vi "2ndStrikerV1.vi"(0 "command\nenum":T11, 1 "Toral de n\natacantes":i32, 2 "Total de robos":u32[](array[numeric]), 3 "N atacantes":u32[](array[numeric]), 4 "AI Parameters":T1={"GotoKick"={"Dist do cone a frente"=150.0, "attacker farback"=1500.0, "Perto"=300.0, "min dist to kick"=150.0, "kick eps"=0.0, "Time to transition"=0.05}, "Attacker"={"CC chute"=0.09, "CC passe"=0.045, "Kick Force"=100.0, "ball-robot Kick"=200.0, "ball-robot Pass"=0.3, "drible\nAttk"=FALSE}, "Defender"={"D max"=1700.0, "Vel p/ robô av"=1000.0, "Kick Force"=100.0, "D atk-def"=0.0, "D farback"=0.0, "drible\ndef"=FALSE, "drible\ngoalie"=FALSE}, "Timeout"={"Field/v in x"=6.0, "Dist Robots"=300, "Dist up in y"=300}, "Pose Striker"={"dist"=200.0, "Numeric"=-4.0, "dist 2"=200.0, "drible\nstriker"=FALSE}, "Dist Stop"=300.0, "D ball out"=200, "D central gap "=150.0, "T pass"=0.0, "Force ++"=0.0, "range kick"=0.0, "Chute alto"=TRUE, "Marcador novo"=TRUE, "drible"=FALSE, "D drible"=300.0, "Versão Striker"=enum."3", "Defesa"=enum."ManMark", "Marcador"=enum."Marcar Segndo mais perigoso", "Receptor passe"=enum."2nd Striker", "Área"=enum."Quadrada"} {"D drible" format="%#_13g"; "D central gap" format="%#_13g"; "Dist Stop" format="%#_13g"; "Pose Striker"."Numeric" format="%#_13g"; "Defender"."Kick Force" format="%#_13g"; "Defender"."Vel p/ robô av" format="%#_13g"; "Attacker"."ball-robot Kick" format="%#_13g"; "Attacker"."Kick Force" format="%#_13g"; "Attacker"."CC passe" format="%#_13g"; "Attacker"."CC chute" format="%#_13g"; "GotoKick"."kick eps" format="%#_13g"; "GotoKick"."min dist to kick" format="%#_13g"; "GotoKick"."Perto" format="%#_13g"; "GotoKick"."attacker farback" format="%#_13g"; "GotoKick"."Dist do cone a frente" format="%#_13g"}, 5 "Robot":T2={"id"=0, "function"=enum."Attacker", "x"=0.0, "y"=0.0, "orientation"=0.0, "v_tangent"=0.0, "v_normal"=0.0, "v_ang"=0.0, "kick_x"=0.0, "kick_z"=0.0, "dribble"=FALSE, "Timestamp"=timestamp(0 s since 1904-01-01), "estimatives"={"est_v_tangent"=0.0, "est_v_normal"=0.0, "est_vx"=0.0, "est_vy"=0.0, "Pos Robot Est"=[]}, "dest_x_kick"=0.0, "dest_y_kick"=0.0, "Gap Coord"=[], "States"=enum."GoToTangent", "Path "=[], "Path  Smooth"=[], "Dest"=[]}, 7 "Field defense":dbl[](array[numeric]), 9 "IA Input":T7={"our_robots"=[], "enemy_robots"=[], "balls"=[], "geometry"={"line_width"=0, "field_length"=0, "field_width"=0, "boundary_width"=0, "referee_width"=0, "goal_width"=0, "goal_depth"=0, "goal_wall_width"=0, "center_circle_radius"=0, "defense_radius"=0, "defense_stretch"=0, "free_kick_from_defense_dist"=0, "penalty_spot_from_field_line_dist"=0, "penalty_line_from_spot_dist"=0}, "IA Judge"={"stage"="", "command"="", "our_goalie_id"=0.0, "enemy_goalie_id"=0.0, "command enum"=enum."Halt", "Time"=enum."Azul"}, "Received Timestamp"=timestamp(0 s since 1904-01-01), "Events"={"Touch"=FALSE, "Ball out"=FALSE, "id touch"=0.0, "Ball out of \nVision"=FALSE, "Ball inside \nGoalie area"=FALSE, "Robot not responding"=FALSE, "Robots responding status"=[1.0, 1.0, 1.0, 1.0, 1.0, 1.0], "Enemy Ball \nPossession"=FALSE, "Pass State"=FALSE, "id end of pass"=0.0, "Kick"=FALSE, "Id ini Possession"=0.0, "Ball Possesion"=FALSE, "Id Possesion"=0.0, "Direct Kick"=FALSE, "2nd Strk Ativo"=FALSE}}, 11 "atacando ao contrário?":bool=TRUE, 12 "Impulso de\ntime elapsed":bool=TRUE, 13 "geometry":T9, 14 "balls":T8[](array[typedef]), 15 "Início de pass state":bool=TRUE) -> (6 "Robot out":T2={"id"=0, "function"=enum."Attacker", "x"=0.0, "y"=0.0, "orientation"=0.0, "v_tangent"=0.0, "v_normal"=0.0, "v_ang"=0.0, "kick_x"=0.0, "kick_z"=0.0, "dribble"=FALSE, "Timestamp"=timestamp(0 s since 1904-01-01), "estimatives"={"est_v_tangent"=0.0, "est_v_normal"=0.0, "est_vx"=0.0, "est_vy"=0.0, "Pos Robot Est"=[]}, "dest_x_kick"=0.0, "dest_y_kick"=0.0, "Gap Coord"=[], "States"=enum."GoToTangent", "Path "=[], "Path  Smooth"=[], "Dest"=[]})   [LabVIEW 2017]
uses:
  Core/AI Robot.ctl
  Functions Enum.ctl
  AttackerStates.ctl
  Path Planning/RRT/PathDests.ctl
  Path Planning/RRT/PathDest.ctl
  Command Enum.ctl
  Core/Field Size.ctl
  Core/AI Ball.ctl
  Core/AI Input.ctl
  Core/AI Judge.ctl
  Util/Events/Events.ctl
  AI Parameters.ctl
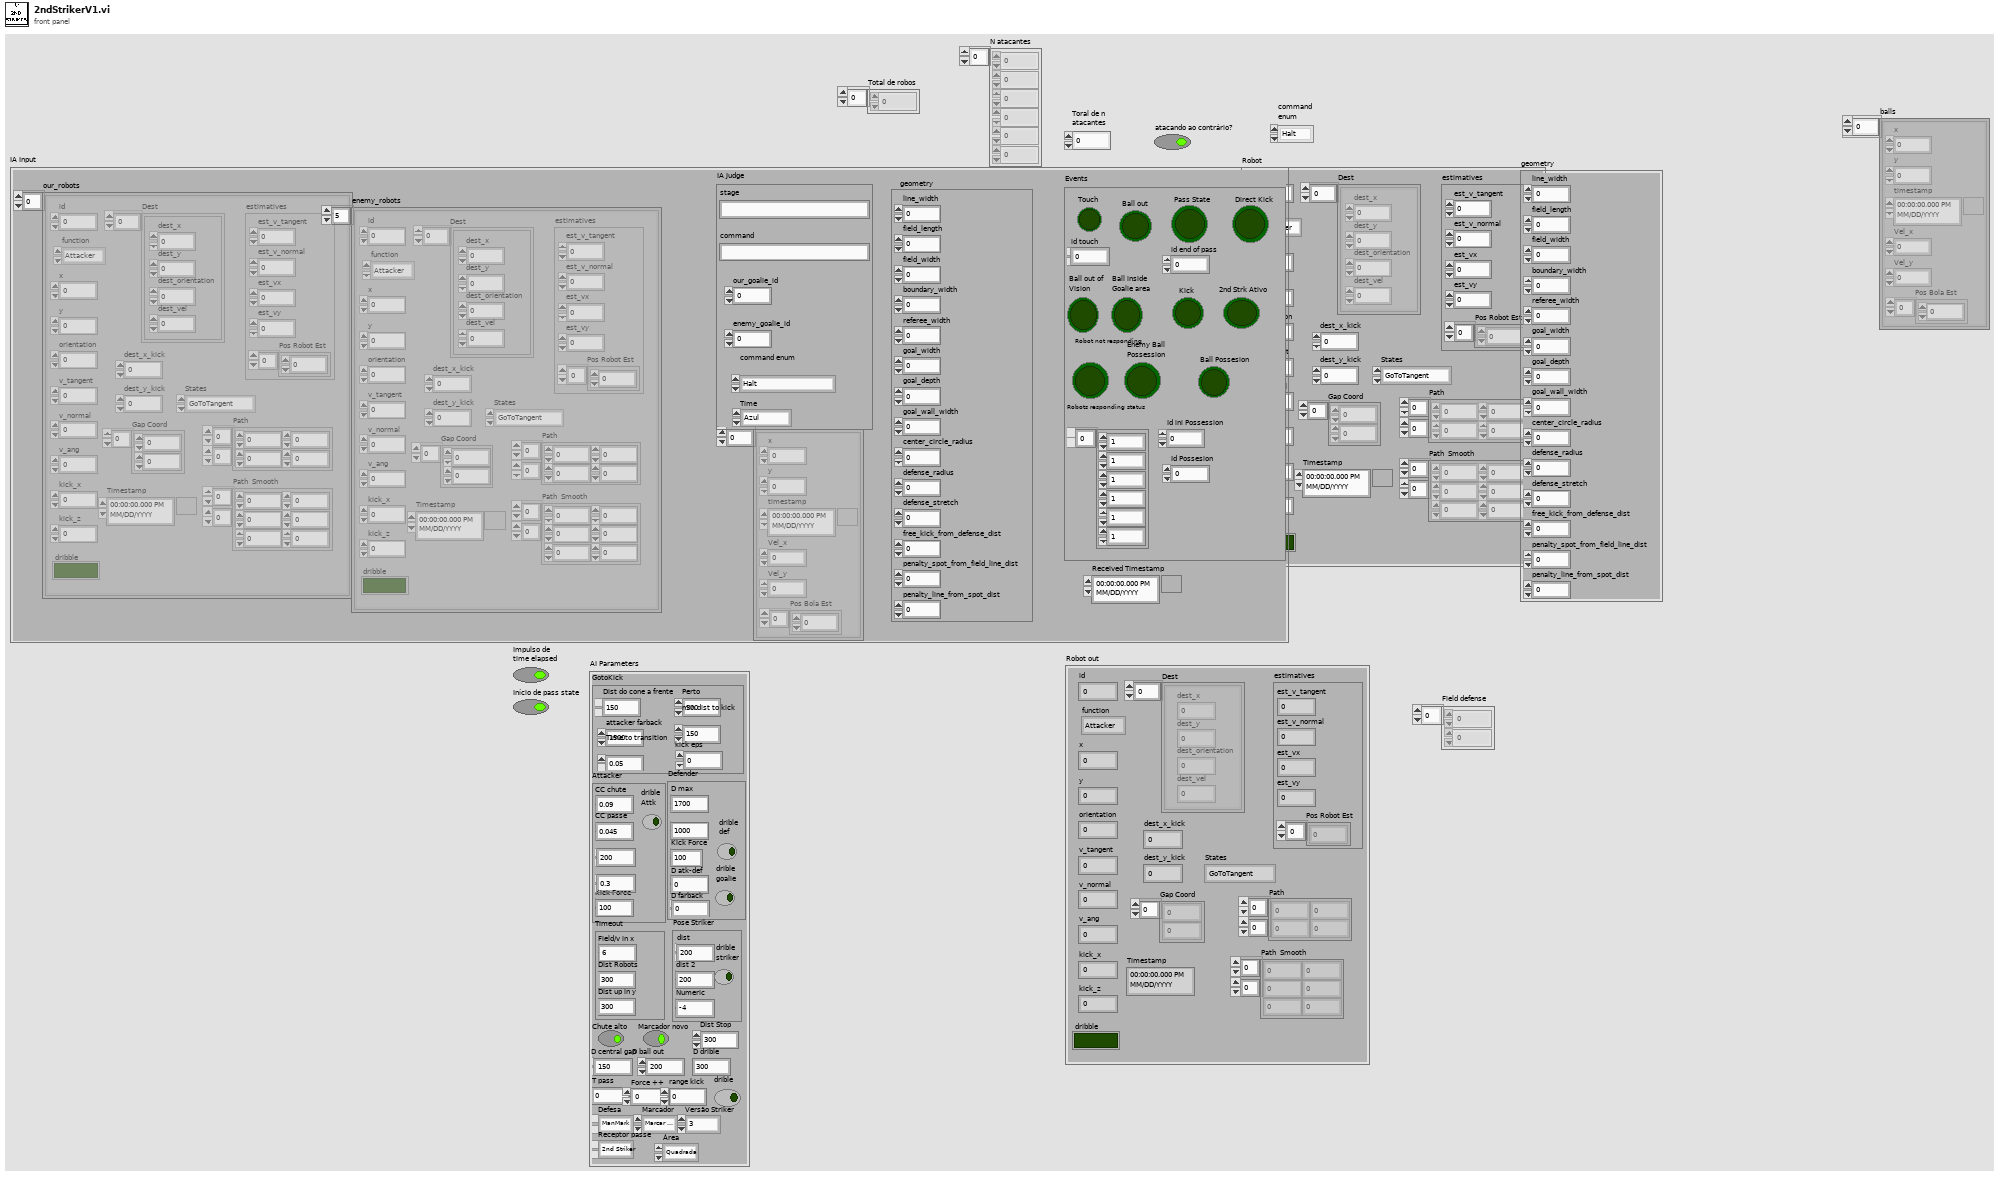
[diagram p1: front panel]
types:
  T1 = typedef "AI Parameters.ctl" = cluster{"GotoKick":cluster{"Dist do cone a frente":dbl, "attacker farback":dbl, "Perto":dbl, "min dist to kick":dbl, "kick eps":dbl, "Time to transition":dbl}, "Attacker":cluster{"CC chute":dbl, "CC passe":dbl, "Kick Force":dbl, "ball-robot Kick":dbl, "ball-robot Pass":dbl, "drible\nAttk":bool}, "Defender":cluster{"D max":dbl, "Vel p/ robô av":dbl, "Kick Force":dbl, "D atk-def":dbl, "D farback":dbl, "drible\ndef":bool, "drible\ngoalie":bool}, "Timeout":cluster{"Field/v in x":dbl, "Dist Robots":u32, "Dist up in y":u32}, "Pose Striker":cluster{"dist":dbl, "Numeric":dbl, "dist 2":dbl, "drible\nstriker":bool}, "Dist Stop":dbl, "D ball out":i32, "D central gap ":dbl, "T pass":dbl, "Force ++":dbl, "range kick":dbl, "Chute alto":bool, "Marcador novo":bool, "drible":bool, "D drible":dbl, "Versão Striker":enum16{"Auto", "3", "2", "1"}, "Defesa":enum16{"ManMark", "Barreira"}, "Marcador":enum16{"Marcar Segndo mais perigoso", "Marcar o mais perigoso"}, "Receptor passe":enum16{"Auto", "2nd Striker", "Striker"}, "Área":enum16{"Quadrada", "Circular"}}
  T2 = typedef "AI Robot.ctl" = cluster{"id":u32, "function":T3, "x":dbl, "y":dbl, "orientation":dbl, "v_tangent":dbl, "v_normal":dbl, "v_ang":dbl, "kick_x":dbl, "kick_z":dbl, "dribble":bool, "Timestamp":timestamp, "estimatives":cluster{"est_v_tangent":dbl, "est_v_normal":dbl, "est_vx":dbl, "est_vy":dbl, "Pos Robot Est":dbl[]}, "dest_x_kick":dbl, "dest_y_kick":dbl, "Gap Coord":dbl[], "States":T4, "Path ":dbl[][], "Path  Smooth":dbl[][], "Dest":T5}
  T3 = typedef "Functions Enum.ctl" = enum16{"2nd Striker", "Attacker", "Goalie", "Defender", "Striker", "Goto 0", "Dummy", "Kicker", "ZigZag 0", "ZigZag 1", "ZigZag 2", "ZigZag 3", "ZigZag 4", "ZigZag 5", "ZigZag 6", "ZigZag 7", "ZigZag 8", ""}
  T4 = typedef "AttackerStates.ctl" = enum16{"Pass", "GoToTangent", "BallGetting", "GoToKick", ""}
  T5 = typedef "PathDests.ctl" = T6[]
  T6 = typedef "PathDest.ctl" = cluster{"dest_x":dbl, "dest_y":dbl, "dest_orientation":dbl, "dest_vel":dbl}
  T7 = typedef "AI Input.ctl" = cluster{"our_robots":T2[], "enemy_robots":T2[], "balls":T8[], "geometry":T9, "IA Judge":T10, "Received Timestamp":timestamp, "Events":T12}
  T8 = typedef "AI Ball.ctl" = cluster{"x":dbl, "y":dbl, "timestamp":timestamp, "Vel_x":dbl, "Vel_y":dbl, "Pos Bola Est":dbl[]}
  T9 = typedef "Field Size.ctl" = cluster{"line_width":u32, "field_length":u32, "field_width":u32, "boundary_width":u32, "referee_width":u32, "goal_width":u32, "goal_depth":u32, "goal_wall_width":u32, "center_circle_radius":u32, "defense_radius":u32, "defense_stretch":u32, "free_kick_from_defense_dist":u32, "penalty_spot_from_field_line_dist":u32, "penalty_line_from_spot_dist":u32}
  T10 = typedef "AI Judge.ctl" = cluster{"stage":string, "command":string, "our_goalie_id":dbl, "enemy_goalie_id":dbl, "command enum":T11, "Time":enum16{"Azul", "Amarelo"}}
  T11 = typedef "Command Enum.ctl" = enum16{"Halt", "Stop", "Force Start", "PKA Normal Start", "Prepare Kickoff Ally", "PKE Normal Start", "Prepare Kickoff Enemy", "Prepare Penalty Ally", "PPA Normal Start", "Prepare Penalty Enemy", "PPE Normal Start", "Direct Free Enemy", "Direct Free Ally", "Indirect Free Enemy", "Indirect Free Ally", "Timeout Enemy", "Timeout Ally", "Goal Enemy", "Goal Ally", "Ball Placement Enemy", "Ball Placement Ally", "Normal Half Time", "Extra Time Break", "Extra Half Time", "None", "Post Game"}
  T12 = typedef "Events.ctl" = cluster{"Touch":bool, "Ball out":bool, "id touch":dbl, "Ball out of \nVision":bool, "Ball inside \nGoalie area":bool, "Robot not responding":bool, "Robots responding status":dbl[], "Enemy Ball \nPossession":bool, "Pass State":bool, "id end of pass":dbl, "Kick":bool, "Id ini Possession":dbl, "Ball Possesion":bool, "Id Possesion":dbl, "Direct Kick":bool, "2nd Strk Ativo":bool}
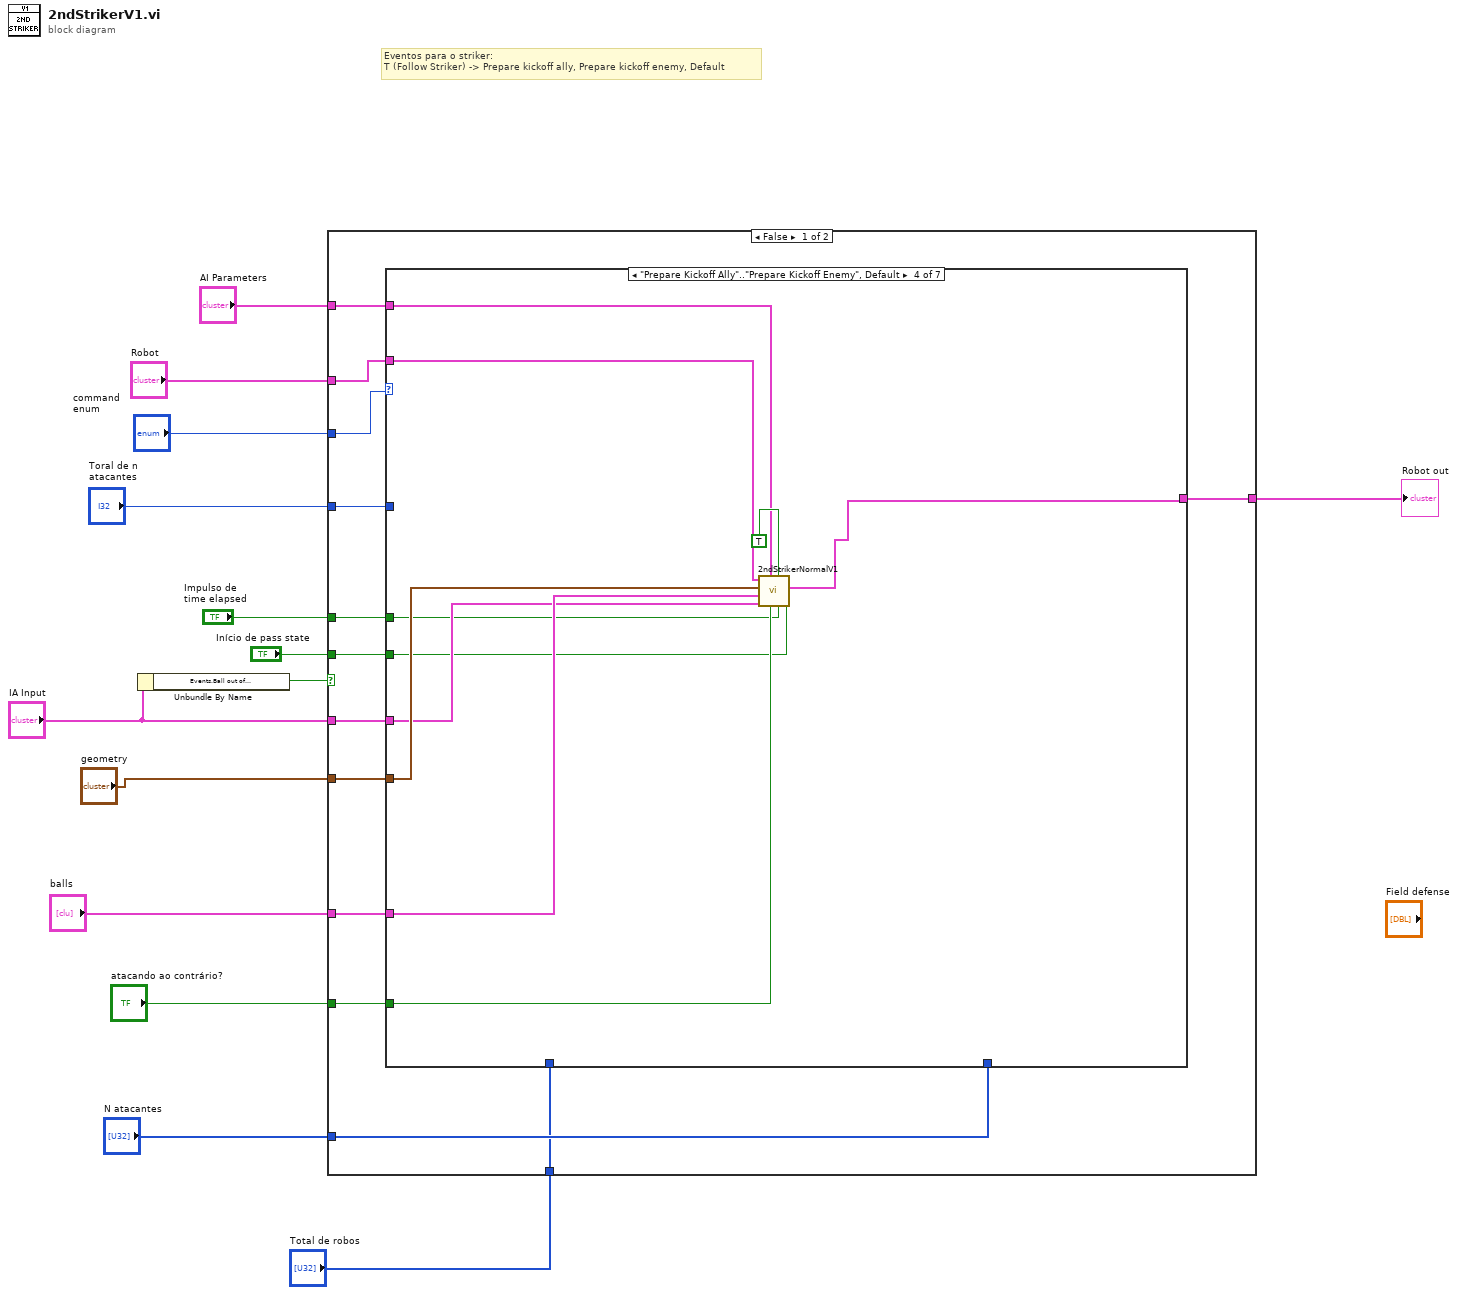
[diagram p0: block diagram]
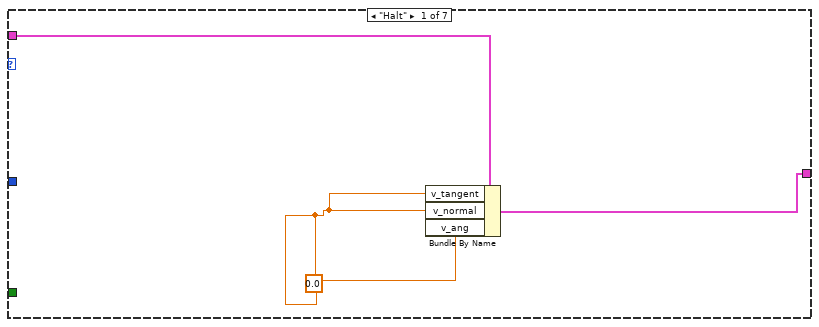
[diagram p2: hidden frame]
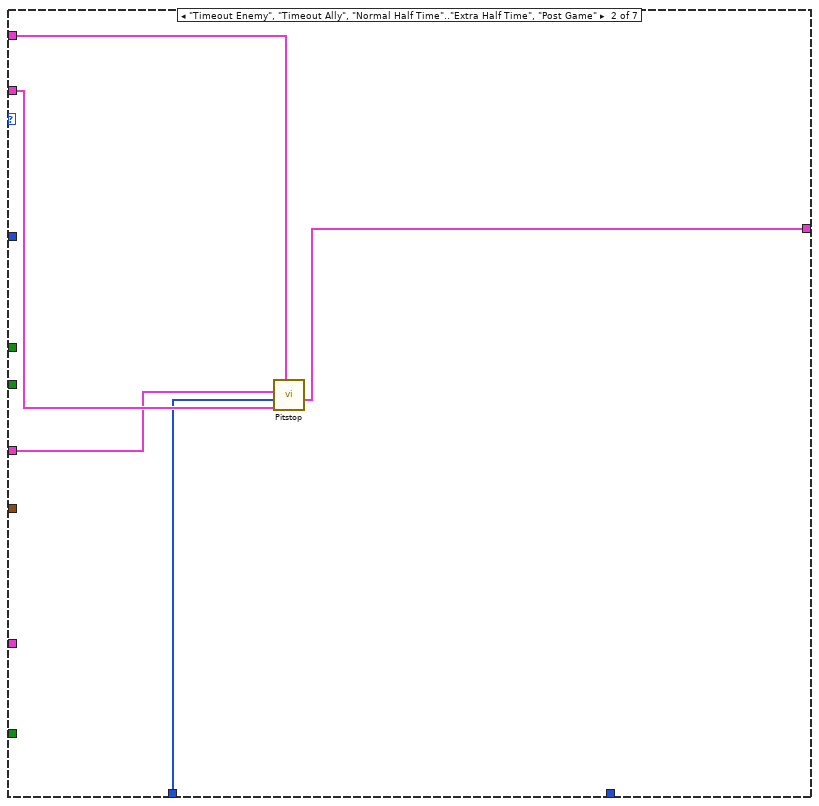
[diagram p3: hidden frame]
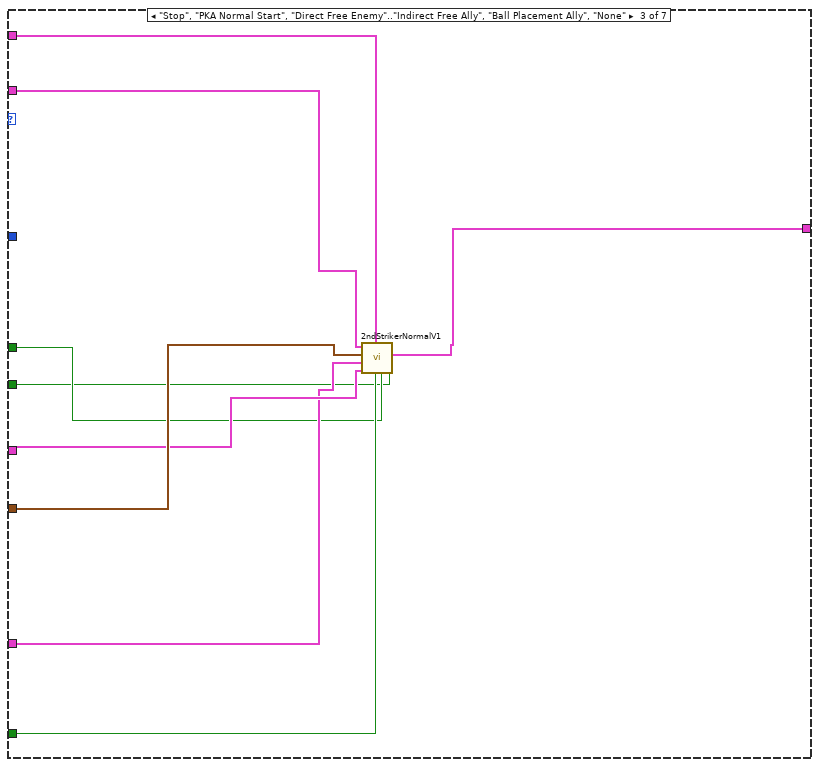
[diagram p4: hidden frame]
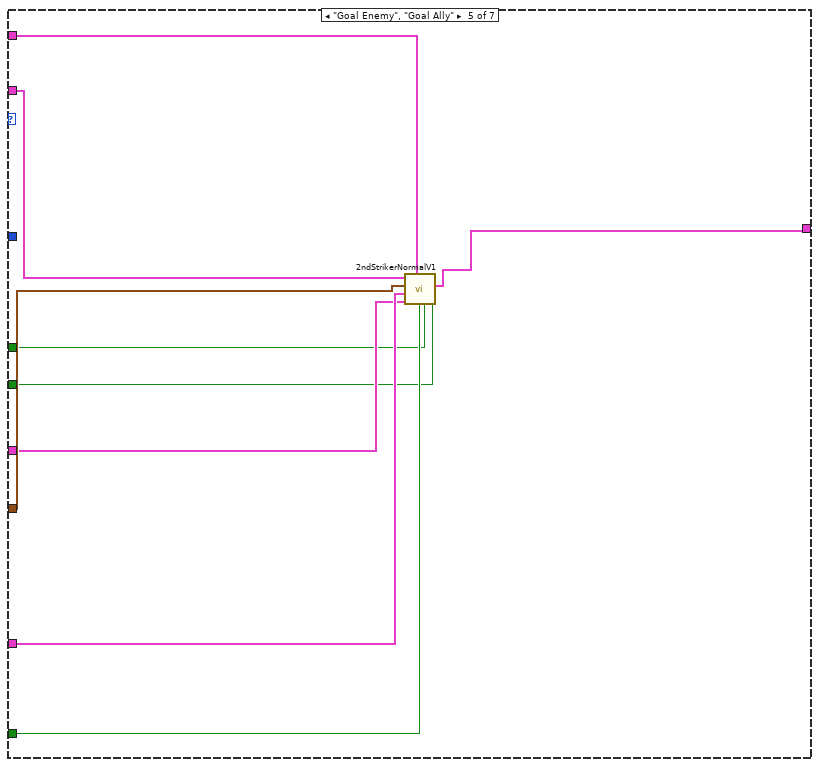
[diagram p5: hidden frame]
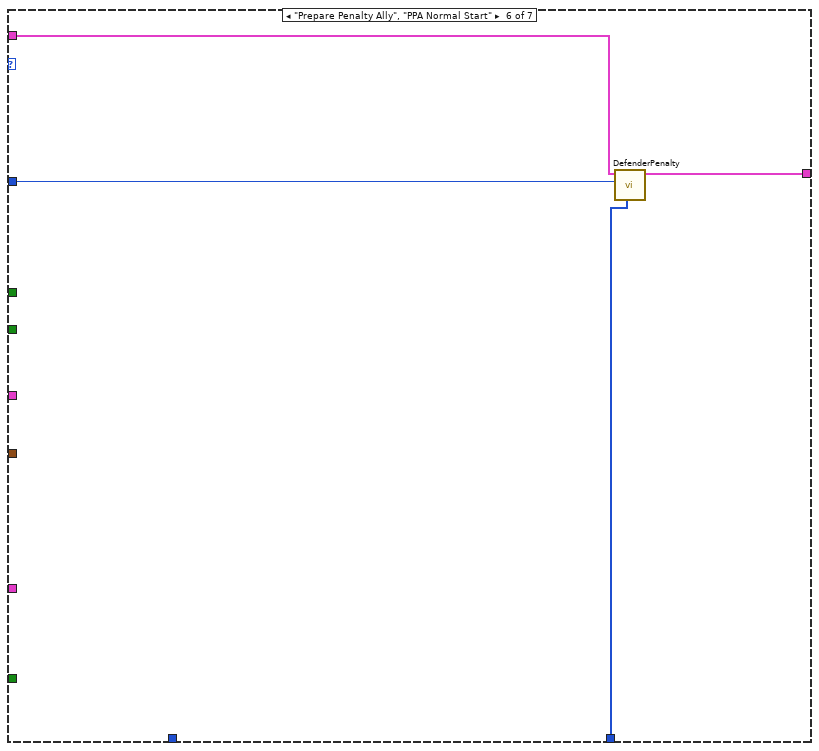
[diagram p6: hidden frame]
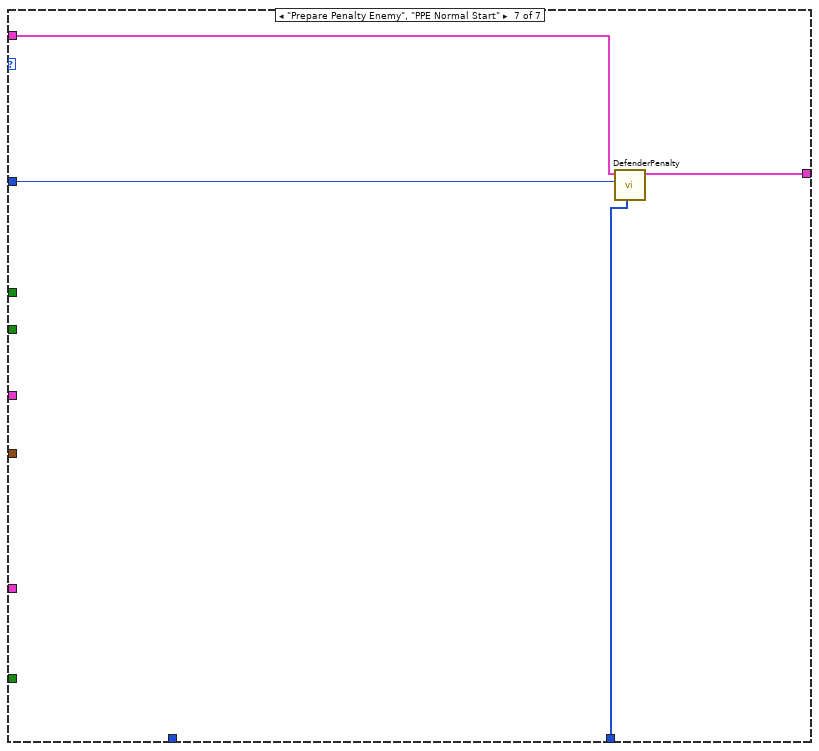
[diagram p7: hidden frame]
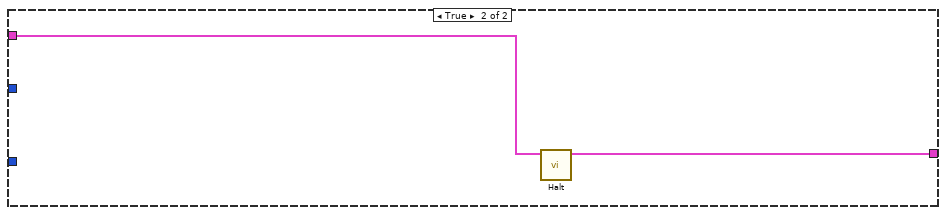
[diagram p8: hidden frame]
diagram:
  # "Eventos para o striker:\nT (Follow Striker) -> Prepare kickoff ally, Prepare kickoff enemy, Default"
  n1 = Unbundle By Name("IA Input") -> ("Events.Ball out of \nVision"=w5:bool)
  n2 = case shown="False" w5 {
    tunnel: "command\nenum" -> [w27 _]
    tunnel: "Robot" -> [w26 w72]
    tunnel: [w25 w73] -> w12
    tunnel: "geometry" -> [w24 _]
    tunnel: "balls" -> [w23 _]
    tunnel: "IA Input" -> [w22 _]
    tunnel: "atacando ao contrário?" -> [w21 _]
    tunnel: "Toral de n\natacantes" -> [w20 _]
    tunnel: "N atacantes" -> [w19 _]
    tunnel: "Total de robos" -> [w18 _]
    tunnel: "AI Parameters" -> [w17 _]
    tunnel: "Impulso de\ntime elapsed" -> [w16 _]
    tunnel: "Início de pass state" -> [w15 _]
    frame False {
      n3 = case shown="\"Prepare Kickoff Ally\"..\"Prepare Kickoff Enemy\", Default" w27 {
        tunnel: w26 -> [w29 w35 w42 w50 w57 w66 w70]
        tunnel: [w28 w32 w44 w53 w63 w67 w71] -> w25
        tunnel: w24 -> [_ _ w41 w51 w62 _ _]
        tunnel: w23 -> [_ _ w39 w49 w61 _ _]
        tunnel: w22 -> [_ w33 w40 w48 w60 _ _]
        tunnel: w21 -> [_ _ w38 w47 w59 _ _]
        tunnel: w20 -> [_ _ _ _ _ w65 w69]
        tunnel: w19 -> [_ _ _ _ _ w64 w68]
        tunnel: w18 -> [_ w34 _ _ _ _ _]
        tunnel: w17 -> [_ w31 w43 w52 w58 _ _]
        tunnel: w16 -> [_ _ w37 w46 w56 _ _]
        tunnel: w15 -> [_ _ w36 w45 w55 _ _]
        frame "Halt" {
          w30 = 0.0
          n4 = Bundle By Name(cluster=w29, "v_tangent"=w30, "v_normal"=w30, "v_ang"=w30) -> (w28:T2)
        }
        frame "Timeout Enemy", "Timeout Ally", "Normal Half Time".."Extra Half Time", "Post Game" {
          n5 = call "Pitstop.vi"("AI Parameters"=w31, "Robot in"=w35, "robos"=w34, "IA State Input"=w33) -> ("Robot out"=w32:T2)  [unwired: 7 in]
        }
        frame "Stop", "PKA Normal Start", "Direct Free Enemy".."Indirect Free Ally", "Ball Placement Ally", "None" {
          n6 = call "2ndStrikerNormalV1.vi"("Início de pass state"=w36, "Impulso de\ntime elapsed"=w37, "atacando ao contrário?"=w38, "AI Parameters"=w43, "IA Input"=w40, "balls"=w39, "Field Size in"=w41, "Robot in"=w42) -> ("Robot out"=w44:T2)  [unwired: 3 in]
        }
        frame "Prepare Kickoff Ally".."Prepare Kickoff Enemy", Default {
          n7 = call "2ndStrikerNormalV1.vi"("Início de pass state"=w45, "Impulso de\ntime elapsed"=w46, "Stop"=TRUE, "atacando ao contrário?"=w47, "AI Parameters"=w52, "IA Input"=w48, "balls"=w49, "Field Size in"=w51, "Robot in"=w50) -> ("Robot out"=w53:T2)  [unwired: 2 in]
        }
        frame "Goal Enemy", "Goal Ally" {
          n8 = call "2ndStrikerNormalV1.vi"("Início de pass state"=w55, "Impulso de\ntime elapsed"=w56, "atacando ao contrário?"=w59, "AI Parameters"=w58, "IA Input"=w60, "balls"=w61, "Field Size in"=w62, "Robot in"=w57) -> ("Robot out"=w63:T2)  [unwired: 3 in]
        }
        frame "Prepare Penalty Ally", "PPA Normal Start" {
          n9 = call "DefenderPenalty.vi"("N atacantes"=w64, "Total de n \natacantes"=w65, "Robot in"=w66) -> ("Robot out"=w67:T2)  [unwired: 8 in]
        }
        frame "Prepare Penalty Enemy", "PPE Normal Start" {
          n10 = call "DefenderPenalty.vi"("N atacantes"=w68, "Total de n \natacantes"=w69, "Robot in"=w70) -> ("Robot out"=w71:T2)  [unwired: 8 in]
        }
      }
    }
    frame True {
      n11 = call "Halt.vi"("Robot in"=w72) -> ("Robot out"=w73:T2)  [unwired: 10 in]
    }
  }
  "Robot out" <- w12
